vi "Auto Filenames.vi"(8 "Fehler (Eingang)":errorcluster, 9 "Flags Cluster":T4={"PDF Optionen (Eingang)"={"PDF Einzelseiten Komponenten"=FALSE, "PDF Einzelseiten Span"=FALSE, "PDF Deckblatt"=FALSE, "PDF öffnen"=FALSE, "Graphik für Messwerte"=FALSE}, "reprocessing"=FALSE, "1. Komponente"=TRUE, "Pfad AutoLIN in"=path "", "File Name LIN in"="", "Pfad LIN in"=path "", "Filename Overrride"=TRUE}, 10 "Zeitstempel":timestamp, 11 "SpanInletClusterArray in":T9[](array[typedef]) {"zusätzliche Zeitdauer Erster Punkt" min=30 step=1 format="%#_5g"; "Zeitdauer Stufen" format="%#_5g"; "Max Fehler" format="%#_5g"; "Anzahl Stufen" format="%#_5g"; "Komponenten"."Komponente 5"."Komponente:" items=["NO (350,3000) LP 191C", "NO2 (150) LP 191C (1of2)", "NO2 (2000) LP 191C (2of2)", "N2O (300) LP 191C (1of2)", "NH3 (300) LP 191C (1of2)", "NH3 (900,3000) LP 191C (2of2)", "HNCO (400) 191C", "H2O% (30) LP 191C", "Formaldehyde (70,500) LP 191C", "CO2 low% (4) LP 191C (2of2)", "CO2% (20) LP 191C (1of2)", "CO (700) LP 191C (1of3)", "CO% (1) LP 191C (2of3)", "Propylene (1000) LP 191C", "Aromatic HC C7 (500) LP 191C", "Ethylene (1000) LP 191C", "CH4 (250) LP 191C (1of2)", "CH4 (5000) LP 191C (2of2)", "Ethane (1000) LP 191C", "Acetylene (1000) LP 191C", "HNO2 (20) 191C", "MeOH (1000) 191C", "CO% (10) LP 191C (3of3)", "Formic Acid (100) 191C", "SO2 (500) LP 191C", "Acetaldehyde (1000) LP 191C", "COS (100) LP 191C", "1,3 butadiene (100) LP 191C", "Oil as Octane (200) LP 191C", "N2O (1000) LP 191C (2of2)", "Propane (200) LP 191C", "NO2 autorange (2000)", "CO autorange (100000)", "CH4 autorange (5000)", "NH3 autorange (3000)", "Temp. Gascell", "Pressure Gascell", "sBeam@2500"]; "Komponenten"."Komponente 5"."Konzentration IST" format="%#.4f"; "Komponenten"."Komponente 5"."Genauigkeit" format="%#.1f"; "Komponenten"."Komponente 4"."Komponente:" items=["NO (350,3000) LP 191C", "NO2 (150) LP 191C (1of2)", "NO2 (2000) LP 191C (2of2)", "N2O (300) LP 191C (1of2)", "NH3 (300) LP 191C (1of2)", "NH3 (900,3000) LP 191C (2of2)", "HNCO (400) 191C", "H2O% (30) LP 191C", "Formaldehyde (70,500) LP 191C", "CO2 low% (4) LP 191C (2of2)", "CO2% (20) LP 191C (1of2)", "CO (700) LP 191C (1of3)", "CO% (1) LP 191C (2of3)", "Propylene (1000) LP 191C", "Aromatic HC C7 (500) LP 191C", "Ethylene (1000) LP 191C", "CH4 (250) LP 191C (1of2)", "CH4 (5000) LP 191C (2of2)", "Ethane (1000) LP 191C", "Acetylene (1000) LP 191C", "HNO2 (20) 191C", "MeOH (1000) 191C", "CO% (10) LP 191C (3of3)", "Formic Acid (100) 191C", "SO2 (500) LP 191C", "Acetaldehyde (1000) LP 191C", "COS (100) LP 191C", "1,3 butadiene (100) LP 191C", "Oil as Octane (200) LP 191C", "N2O (1000) LP 191C (2of2)", "Propane (200) LP 191C", "NO2 autorange (2000)", "CO autorange (100000)", "CH4 autorange (5000)", "NH3 autorange (3000)", "Temp. Gascell", "Pressure Gascell", "sBeam@2500"]; "Komponenten"."Komponente 4"."Konzentration IST" format="%#.4f"; "Komponenten"."Komponente 4"."Genauigkeit" format="%#.1f"; "Komponenten"."Komponente 3"."Komponente:" items=["NO (350,3000) LP 191C", "NO2 (150) LP 191C (1of2)", "NO2 (2000) LP 191C (2of2)", "N2O (300) LP 191C (1of2)", "NH3 (300) LP 191C (1of2)", "NH3 (900,3000) LP 191C (2of2)", "HNCO (400) 191C", "H2O% (30) LP 191C", "Formaldehyde (70,500) LP 191C", "CO2 low% (4) LP 191C (2of2)", "CO2% (20) LP 191C (1of2)", "CO (700) LP 191C (1of3)", "CO% (1) LP 191C (2of3)", "Propylene (1000) LP 191C", "Aromatic HC C7 (500) LP 191C", "Ethylene (1000) LP 191C", "CH4 (250) LP 191C (1of2)", "CH4 (5000) LP 191C (2of2)", "Ethane (1000) LP 191C", "Acetylene (1000) LP 191C", "HNO2 (20) 191C", "MeOH (1000) 191C", "CO% (10) LP 191C (3of3)", "Formic Acid (100) 191C", "SO2 (500) LP 191C", "Acetaldehyde (1000) LP 191C", "COS (100) LP 191C", "1,3 butadiene (100) LP 191C", "Oil as Octane (200) LP 191C", "N2O (1000) LP 191C (2of2)", "Propane (200) LP 191C", "NO2 autorange (2000)", "CO autorange (100000)", "CH4 autorange (5000)", "NH3 autorange (3000)", "Temp. Gascell", "Pressure Gascell", "sBeam@2500"]; "Komponenten"."Komponente 3"."Konzentration IST" format="%#.4f"; "Komponenten"."Komponente 3"."Genauigkeit" format="%#.1f"; "Komponenten"."Komponente 2"."Komponente:" items=["NO (350,3000) LP 191C", "NO2 (150) LP 191C (1of2)", "NO2 (2000) LP 191C (2of2)", "N2O (300) LP 191C (1of2)", "NH3 (300) LP 191C (1of2)", "NH3 (900,3000) LP 191C (2of2)", "HNCO (400) 191C", "H2O% (30) LP 191C", "Formaldehyde (70,500) LP 191C", "CO2 low% (4) LP 191C (2of2)", "CO2% (20) LP 191C (1of2)", "CO (700) LP 191C (1of3)", "CO% (1) LP 191C (2of3)", "Propylene (1000) LP 191C", "Aromatic HC C7 (500) LP 191C", "Ethylene (1000) LP 191C", "CH4 (250) LP 191C (1of2)", "CH4 (5000) LP 191C (2of2)", "Ethane (1000) LP 191C", "Acetylene (1000) LP 191C", "HNO2 (20) 191C", "MeOH (1000) 191C", "CO% (10) LP 191C (3of3)", "Formic Acid (100) 191C", "SO2 (500) LP 191C", "Acetaldehyde (1000) LP 191C", "COS (100) LP 191C", "1,3 butadiene (100) LP 191C", "Oil as Octane (200) LP 191C", "N2O (1000) LP 191C (2of2)", "Propane (200) LP 191C", "NO2 autorange (2000)", "CO autorange (100000)", "CH4 autorange (5000)", "NH3 autorange (3000)", "Temp. Gascell", "Pressure Gascell", "sBeam@2500"]; "Komponenten"."Komponente 2"."Konzentration IST" format="%#.4f"; "Komponenten"."Komponente 2"."Genauigkeit" format="%#.1f"; "Komponenten"."Komponente 1"."Komponente:" items=["NO (350,3000) LP 191C", "NO2 (150) LP 191C (1of2)", "NO2 (2000) LP 191C (2of2)", "N2O (300) LP 191C (1of2)", "NH3 (300) LP 191C (1of2)", "NH3 (900,3000) LP 191C (2of2)", "HNCO (400) 191C", "H2O% (30) LP 191C", "Formaldehyde (70,500) LP 191C", "CO2 low% (4) LP 191C (2of2)", "CO2% (20) LP 191C (1of2)", "CO (700) LP 191C (1of3)", "CO% (1) LP 191C (2of3)", "Propylene (1000) LP 191C", "Aromatic HC C7 (500) LP 191C", "Ethylene (1000) LP 191C", "CH4 (250) LP 191C (1of2)", "CH4 (5000) LP 191C (2of2)", "Ethane (1000) LP 191C", "Acetylene (1000) LP 191C", "HNO2 (20) 191C", "MeOH (1000) 191C", "CO% (10) LP 191C (3of3)", "Formic Acid (100) 191C", "SO2 (500) LP 191C", "Acetaldehyde (1000) LP 191C", "COS (100) LP 191C", "1,3 butadiene (100) LP 191C", "Oil as Octane (200) LP 191C", "N2O (1000) LP 191C (2of2)", "Propane (200) LP 191C", "NO2 autorange (2000)", "CO autorange (100000)", "CH4 autorange (5000)", "NH3 autorange (3000)", "Temp. Gascell", "Pressure Gascell", "sBeam@2500"]; "Komponenten"."Komponente 1"."Konzentration IST" format="%#.4f"; "Komponenten"."Komponente 1"."Genauigkeit" format="%#.1f"; "Ablaufdatum" format="%<%d.%m.%Y>T"; "Gasflasche" items=["----"=10000, "IAG NH3 3000"=0, "IAG NH3 200"=1, "IAG NH3 2000"=2, "IAG MG"=3, "IAG O2"=4]}) -> (0 "Fehler (Ausgang)":errorcluster, 1 "LogInfo-Cluster":T6 {"Gasflasche" items=["----"=10000, "IAG NH3 3000"=0, "IAG NH3 200"=1, "IAG NH3 2000"=2, "IAG MG"=3, "IAG O2"=4]}, 2 "Pfad LIN Cluster":cluster{"Pfad LIN SPAN":T1, "Pfad LIN":path}, 3 "SpanInletClusterArray out":T9[](array[typedef]) {"zusätzliche Zeitdauer Erster Punkt" min=30 step=1 format="%#_5g"; "Zeitdauer Stufen" format="%#_5g"; "Max Fehler" format="%#_5g"; "Anzahl Stufen" format="%#_5g"; "Komponenten"."Komponente 5"."Komponente:" items=["NO (350,3000) LP 191C", "NO2 (150) LP 191C (1of2)", "NO2 (2000) LP 191C (2of2)", "N2O (300) LP 191C (1of2)", "NH3 (300) LP 191C (1of2)", "NH3 (900,3000) LP 191C (2of2)", "HNCO (400) 191C", "H2O% (30) LP 191C", "Formaldehyde (70,500) LP 191C", "CO2 low% (4) LP 191C (2of2)", "CO2% (20) LP 191C (1of2)", "CO (700) LP 191C (1of3)", "CO% (1) LP 191C (2of3)", "Propylene (1000) LP 191C", "Aromatic HC C7 (500) LP 191C", "Ethylene (1000) LP 191C", "CH4 (250) LP 191C (1of2)", "CH4 (5000) LP 191C (2of2)", "Ethane (1000) LP 191C", "Acetylene (1000) LP 191C", "HNO2 (20) 191C", "MeOH (1000) 191C", "CO% (10) LP 191C (3of3)", "Formic Acid (100) 191C", "SO2 (500) LP 191C", "Acetaldehyde (1000) LP 191C", "COS (100) LP 191C", "1,3 butadiene (100) LP 191C", "Oil as Octane (200) LP 191C", "N2O (1000) LP 191C (2of2)", "Propane (200) LP 191C", "NO2 autorange (2000)", "CO autorange (100000)", "CH4 autorange (5000)", "NH3 autorange (3000)", "Temp. Gascell", "Pressure Gascell", "sBeam@2500"]; "Komponenten"."Komponente 5"."Konzentration IST" format="%#.4f"; "Komponenten"."Komponente 5"."Genauigkeit" format="%#.1f"; "Komponenten"."Komponente 4"."Komponente:" items=["NO (350,3000) LP 191C", "NO2 (150) LP 191C (1of2)", "NO2 (2000) LP 191C (2of2)", "N2O (300) LP 191C (1of2)", "NH3 (300) LP 191C (1of2)", "NH3 (900,3000) LP 191C (2of2)", "HNCO (400) 191C", "H2O% (30) LP 191C", "Formaldehyde (70,500) LP 191C", "CO2 low% (4) LP 191C (2of2)", "CO2% (20) LP 191C (1of2)", "CO (700) LP 191C (1of3)", "CO% (1) LP 191C (2of3)", "Propylene (1000) LP 191C", "Aromatic HC C7 (500) LP 191C", "Ethylene (1000) LP 191C", "CH4 (250) LP 191C (1of2)", "CH4 (5000) LP 191C (2of2)", "Ethane (1000) LP 191C", "Acetylene (1000) LP 191C", "HNO2 (20) 191C", "MeOH (1000) 191C", "CO% (10) LP 191C (3of3)", "Formic Acid (100) 191C", "SO2 (500) LP 191C", "Acetaldehyde (1000) LP 191C", "COS (100) LP 191C", "1,3 butadiene (100) LP 191C", "Oil as Octane (200) LP 191C", "N2O (1000) LP 191C (2of2)", "Propane (200) LP 191C", "NO2 autorange (2000)", "CO autorange (100000)", "CH4 autorange (5000)", "NH3 autorange (3000)", "Temp. Gascell", "Pressure Gascell", "sBeam@2500"]; "Komponenten"."Komponente 4"."Konzentration IST" format="%#.4f"; "Komponenten"."Komponente 4"."Genauigkeit" format="%#.1f"; "Komponenten"."Komponente 3"."Komponente:" items=["NO (350,3000) LP 191C", "NO2 (150) LP 191C (1of2)", "NO2 (2000) LP 191C (2of2)", "N2O (300) LP 191C (1of2)", "NH3 (300) LP 191C (1of2)", "NH3 (900,3000) LP 191C (2of2)", "HNCO (400) 191C", "H2O% (30) LP 191C", "Formaldehyde (70,500) LP 191C", "CO2 low% (4) LP 191C (2of2)", "CO2% (20) LP 191C (1of2)", "CO (700) LP 191C (1of3)", "CO% (1) LP 191C (2of3)", "Propylene (1000) LP 191C", "Aromatic HC C7 (500) LP 191C", "Ethylene (1000) LP 191C", "CH4 (250) LP 191C (1of2)", "CH4 (5000) LP 191C (2of2)", "Ethane (1000) LP 191C", "Acetylene (1000) LP 191C", "HNO2 (20) 191C", "MeOH (1000) 191C", "CO% (10) LP 191C (3of3)", "Formic Acid (100) 191C", "SO2 (500) LP 191C", "Acetaldehyde (1000) LP 191C", "COS (100) LP 191C", "1,3 butadiene (100) LP 191C", "Oil as Octane (200) LP 191C", "N2O (1000) LP 191C (2of2)", "Propane (200) LP 191C", "NO2 autorange (2000)", "CO autorange (100000)", "CH4 autorange (5000)", "NH3 autorange (3000)", "Temp. Gascell", "Pressure Gascell", "sBeam@2500"]; "Komponenten"."Komponente 3"."Konzentration IST" format="%#.4f"; "Komponenten"."Komponente 3"."Genauigkeit" format="%#.1f"; "Komponenten"."Komponente 2"."Komponente:" items=["NO (350,3000) LP 191C", "NO2 (150) LP 191C (1of2)", "NO2 (2000) LP 191C (2of2)", "N2O (300) LP 191C (1of2)", "NH3 (300) LP 191C (1of2)", "NH3 (900,3000) LP 191C (2of2)", "HNCO (400) 191C", "H2O% (30) LP 191C", "Formaldehyde (70,500) LP 191C", "CO2 low% (4) LP 191C (2of2)", "CO2% (20) LP 191C (1of2)", "CO (700) LP 191C (1of3)", "CO% (1) LP 191C (2of3)", "Propylene (1000) LP 191C", "Aromatic HC C7 (500) LP 191C", "Ethylene (1000) LP 191C", "CH4 (250) LP 191C (1of2)", "CH4 (5000) LP 191C (2of2)", "Ethane (1000) LP 191C", "Acetylene (1000) LP 191C", "HNO2 (20) 191C", "MeOH (1000) 191C", "CO% (10) LP 191C (3of3)", "Formic Acid (100) 191C", "SO2 (500) LP 191C", "Acetaldehyde (1000) LP 191C", "COS (100) LP 191C", "1,3 butadiene (100) LP 191C", "Oil as Octane (200) LP 191C", "N2O (1000) LP 191C (2of2)", "Propane (200) LP 191C", "NO2 autorange (2000)", "CO autorange (100000)", "CH4 autorange (5000)", "NH3 autorange (3000)", "Temp. Gascell", "Pressure Gascell", "sBeam@2500"]; "Komponenten"."Komponente 2"."Konzentration IST" format="%#.4f"; "Komponenten"."Komponente 2"."Genauigkeit" format="%#.1f"; "Komponenten"."Komponente 1"."Komponente:" items=["NO (350,3000) LP 191C", "NO2 (150) LP 191C (1of2)", "NO2 (2000) LP 191C (2of2)", "N2O (300) LP 191C (1of2)", "NH3 (300) LP 191C (1of2)", "NH3 (900,3000) LP 191C (2of2)", "HNCO (400) 191C", "H2O% (30) LP 191C", "Formaldehyde (70,500) LP 191C", "CO2 low% (4) LP 191C (2of2)", "CO2% (20) LP 191C (1of2)", "CO (700) LP 191C (1of3)", "CO% (1) LP 191C (2of3)", "Propylene (1000) LP 191C", "Aromatic HC C7 (500) LP 191C", "Ethylene (1000) LP 191C", "CH4 (250) LP 191C (1of2)", "CH4 (5000) LP 191C (2of2)", "Ethane (1000) LP 191C", "Acetylene (1000) LP 191C", "HNO2 (20) 191C", "MeOH (1000) 191C", "CO% (10) LP 191C (3of3)", "Formic Acid (100) 191C", "SO2 (500) LP 191C", "Acetaldehyde (1000) LP 191C", "COS (100) LP 191C", "1,3 butadiene (100) LP 191C", "Oil as Octane (200) LP 191C", "N2O (1000) LP 191C (2of2)", "Propane (200) LP 191C", "NO2 autorange (2000)", "CO autorange (100000)", "CH4 autorange (5000)", "NH3 autorange (3000)", "Temp. Gascell", "Pressure Gascell", "sBeam@2500"]; "Komponenten"."Komponente 1"."Konzentration IST" format="%#.4f"; "Komponenten"."Komponente 1"."Genauigkeit" format="%#.1f"; "Ablaufdatum" format="%<%d.%m.%Y>T"; "Gasflasche" items=["----"=10000, "IAG NH3 3000"=0, "IAG NH3 200"=1, "IAG NH3 2000"=2, "IAG MG"=3, "IAG O2"=4]}, 4 "File Name LIN":T3, 5 "Span_Name":string, 6 "File Name EPA":T3, 7 "File Names":T5)   [LabVIEW 2020, in "Linearisierung v2.lvlib" / "SpanEinstellungen.lvlib"]
uses:
  SpanEinstellungen.lvlib
  Visualisierungs Elemente/String - Eingabefeld.ctl
  SpanInletCluster.ctl
  Seiten/System Einstellungen V2/Konfig Gasflasche.ctl
  Seiten/System Einstellungen V2/Analysatoren.ctl
  Seiten/System Einstellungen V2/Gasflasche Auswahl.ctl
  Komponentencluster mit Formel.ctl
  Komponentenauswahl mit Formel.ctl
  Einheit.ctl
  Seiten/System Einstellungen V2/Traegergas.ctl
  ErrorLogInfoCluster.ctl
  Visualisierungs Elemente/String - Ausgabefeld.ctl
  PDF Optionen.ctl
  Visualisierungs Elemente/Pfad-Eingabefeld.ctl
  Aktion FGV Spans abarbeiten.ctl
  Aktion FGV Post Processing.ctl
  Allgemein/allgemeine Sub-VIs.lvlib
  Seiten/System Einstellungen V2/System Einstellungen V2.lvlib
panel:
  out "Deckblatt LIN":string
  out "Deckblatt EPA":string
  # "sec"
  # "%"
  # "sec"
  # "Komponente"
  # "Formel"
  # "Konzentration"
  # "Einheit"
  # "Genauigkeit [%]"
  # "sec"
  # "%"
  # "sec"
  # "Komponente"
  # "Formel"
  # "Konzentration"
  # "Einheit"
  # "Genauigkeit [%]"
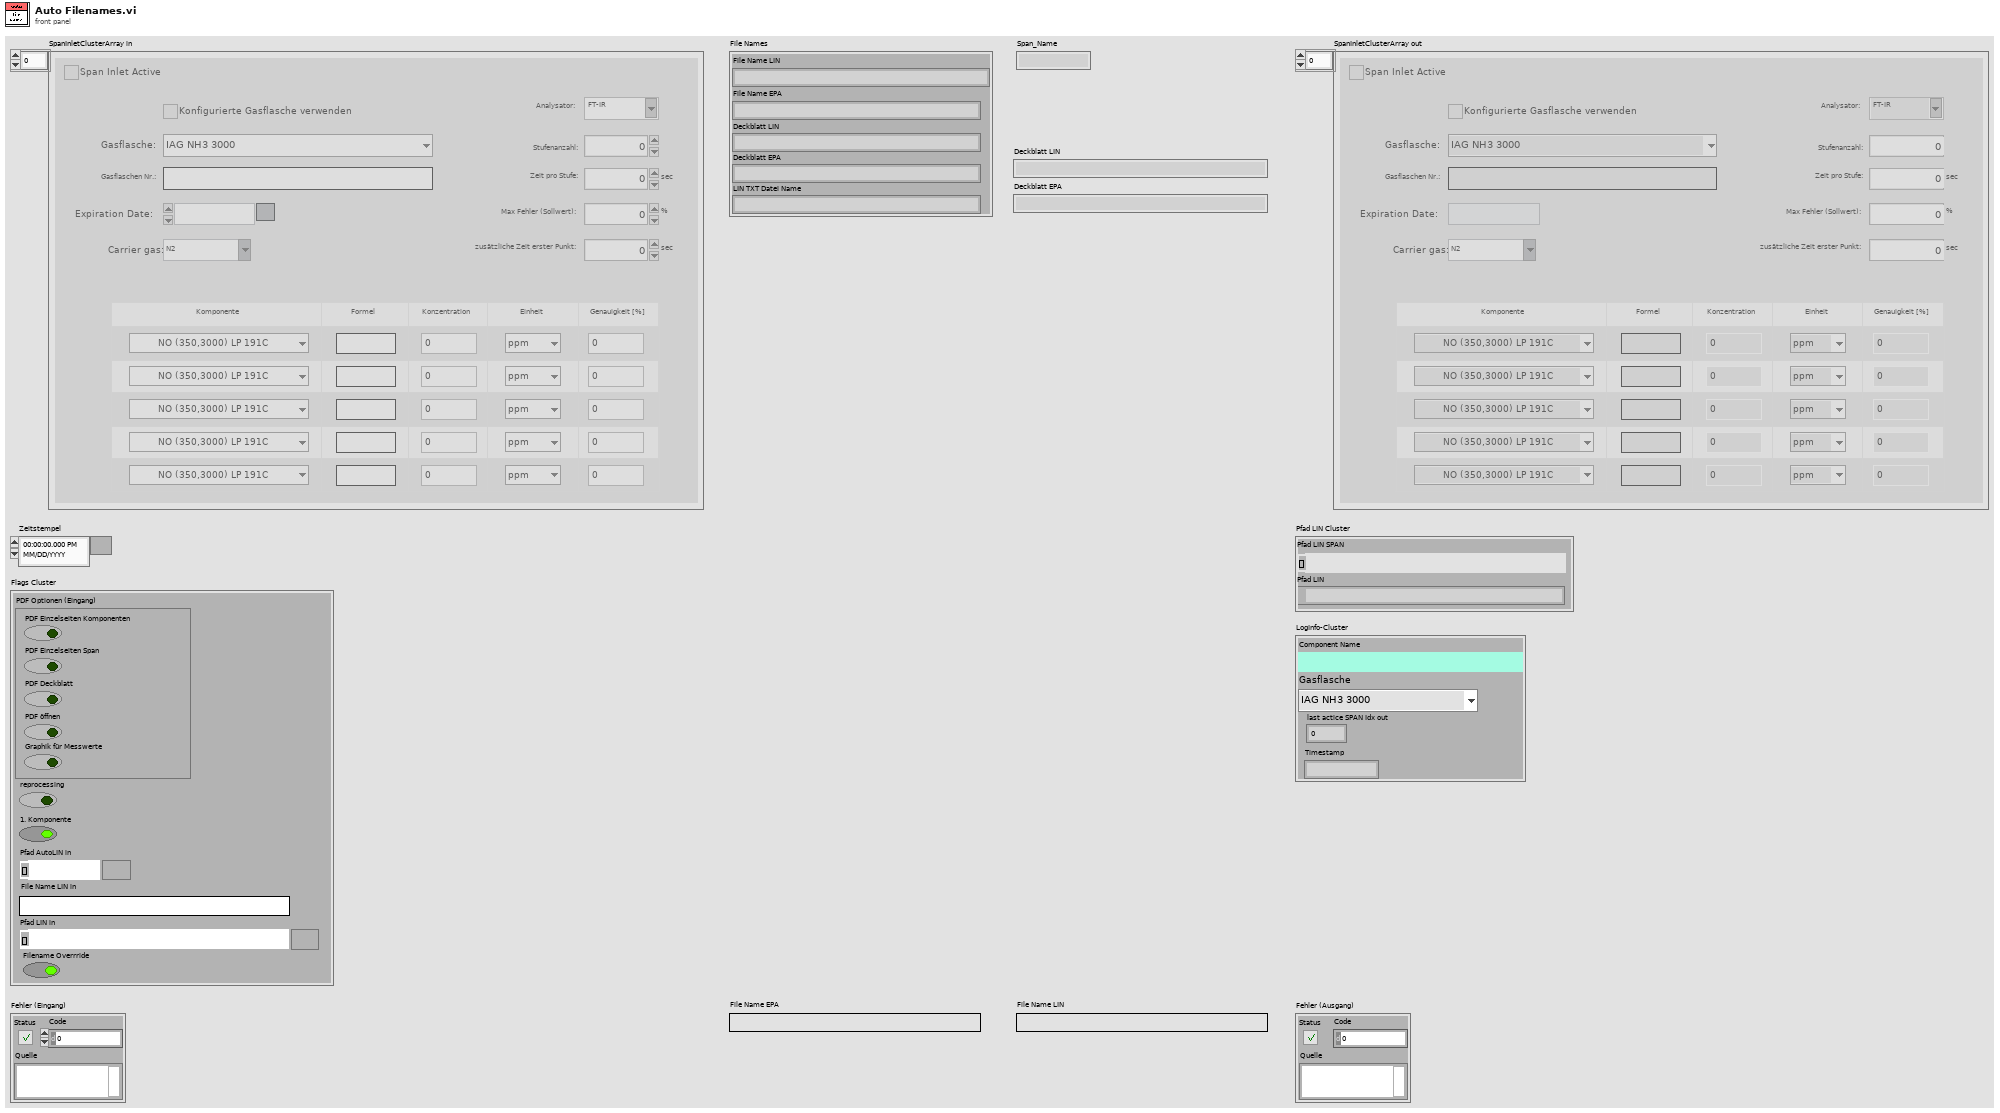
[diagram p1: front panel]
types:
  T1 = typedef "Pfad-Eingabefeld.ctl" = path
  T2 = typedef "Linearisierung v2.lvlib/SpanEinstellungen.lvlib/PDF Optionen.ctl" = cluster{"PDF Einzelseiten Komponenten":bool, "PDF Einzelseiten Span":bool, "PDF Deckblatt":bool, "PDF öffnen":bool, "Graphik für Messwerte":bool}
  T3 = typedef "String - Eingabefeld.ctl" = string
  T4 = cluster{"PDF Optionen (Eingang)":T2, "reprocessing":bool, "1. Komponente":bool, "Pfad AutoLIN in":T1, "File Name LIN in":T3, "Pfad LIN in":T1, "Filename Overrride":bool}
  T5 = cluster{"File Name LIN":string, "File Name EPA":string, "Deckblatt LIN":string, "Deckblatt EPA":string, "LIN TXT Datei Name":string}
  T6 = typedef "Linearisierung v2.lvlib/SpanEinstellungen.lvlib/ErrorLogInfoCluster.ctl" = cluster{"Component Name":T7, "Gasflasche":T8, "last actice SPAN Idx out":i32, "Timestamp":string}
  T7 = typedef "String - Ausgabefeld.ctl" = string
  T8 = typedef "System Einstellungen V2.lvlib/Gasflasche Auswahl.ctl" = u16
  T9 = typedef "Linearisierung v2.lvlib/SpanEinstellungen.lvlib/SpanInletCluster.ctl" = cluster{"Span Inlet Active":T10, "Analysator":T11, "Konfig Gasflasche":T10, "Gasflasche":T8, "Gasflaschen Nr.:":string, "Ablaufdatum":timestamp, "Komponenten":T12, "Zeitdauer Stufen":sgl, "Max Fehler":sgl, "Anzahl Stufen":sgl, "Trägergas":T15, "zusätzliche Zeitdauer Erster Punkt":sgl}
  T10 = typedef "System Einstellungen V2.lvlib/Konfig Gasflasche.ctl" = bool
  T11 = typedef "System Einstellungen V2.lvlib/Analysatoren.ctl" = string
  T12 = typedef "Linearisierung v2.lvlib/SpanEinstellungen.lvlib/Komponentencluster mit Formel.ctl" = cluster{"Komponente 1":T13, "Komponente 2":T13, "Komponente 3":T13, "Komponente 4":T13, "Komponente 5":T13}
  T13 = typedef "Linearisierung v2.lvlib/SpanEinstellungen.lvlib/Komponentenauswahl mit Formel.ctl" = cluster{"Komponente:":u16, "Summenformel":T3, "Konzentration IST":dbl, "Einheit":T14, "Genauigkeit":dbl}
  T14 = typedef "Linearisierung v2.lvlib/SpanEinstellungen.lvlib/Einheit.ctl" = enum16{"ppm", "%"}
  T15 = typedef "System Einstellungen V2.lvlib/Traegergas.ctl" = string
  T16 = typedef "Linearisierung v2.lvlib/SpanEinstellungen.lvlib/Aktion FGV Spans abarbeiten.ctl" = enum16{"lesen", "idle", "start", "next", "comp", "init", "running", "abort"}
  T17 = typedef "Linearisierung v2.lvlib/SpanEinstellungen.lvlib/Aktion FGV Post Processing.ctl" = enum16{"lesen", "set ref", "init", "reset", "enable", "disable", "filenames", "active", "comp", "filename index", "next", "first", "abort", "show", "same"}
  T18 = typedef "Linearisierung v2.lvlib/SpanEinstellungen.lvlib/Postprocessing_Running_Indices.ctl" = cluster{"active postprocessing SPAN":i32, "active postprocessing SPAN Component":i32, "active postprocessing index":i32}
  T19 = cluster{"active Index Cluster out":T18, "last postprocessing SPAN ":bool}
  T20 = cluster{"Component Name":T7, "Compnent Nr":u16, "Formelname(n)":string}
  T21 = cluster{"File Name LIN":string, "File Name EPA":string, "MG":bool}
  T22 = cluster{"Component Name":T7, "Gasflasche":T8, "active postprocessing SPAN":i32, "date/time string":string}
  T23 = cluster{"File Name LIN in":T3, "File Name LIN in":T3, string, string, "File Name LIN":string}
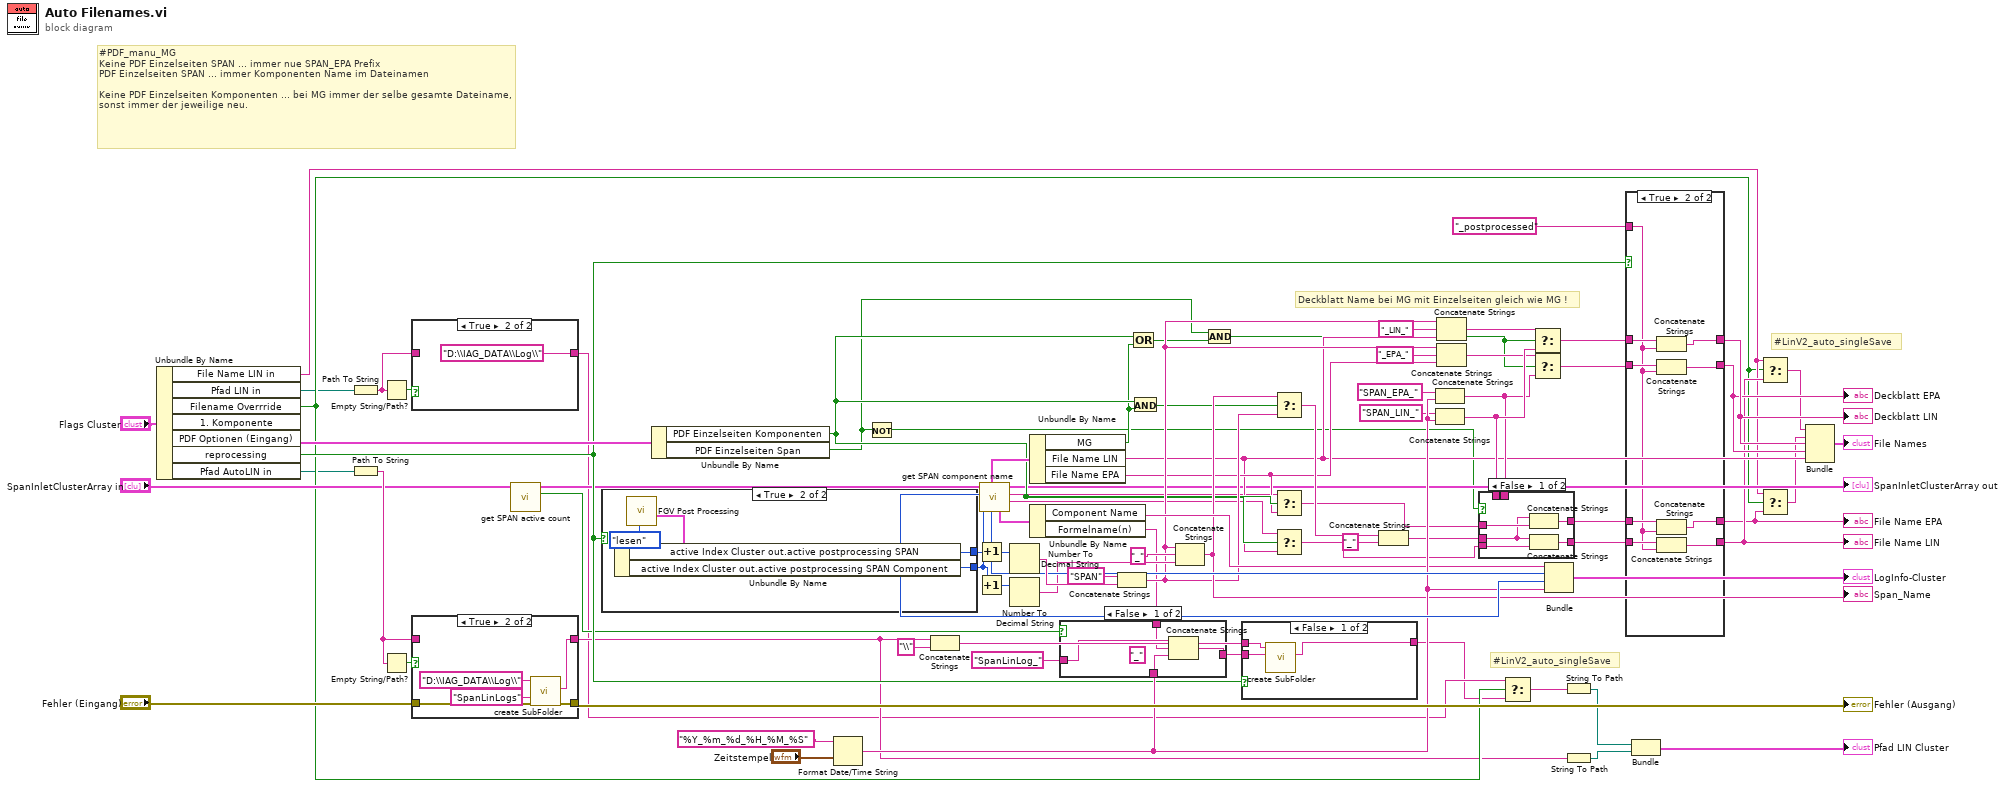
[diagram p0: block diagram]
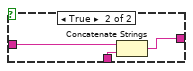
[diagram p4: hidden frame]
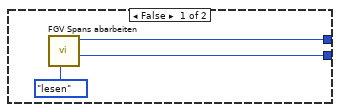
[diagram p6: hidden frame]
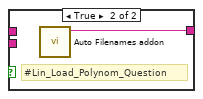
[diagram p7: hidden frame]
diagram:
  # "#LinV2_auto_singleSave"
  # "#LinV2_auto_singleSave"
  # "Deckblatt Name bei MG mit Einzelseiten gleich wie MG !"
  # "#PDF_manu_MG\nKeine PDF Einzelseiten SPAN ... immer nue SPAN_EPA Prefix\nPDF Einzelseiten SPAN ... immer Komponenten Name im Dateinamen\n\nKeine PDF Einzelseiten Komponenten ... bei MG immer der selbe gesamte Dateiname, sonst immer der jeweilige neu."
  n1 = Unbundle By Name("Flags Cluster") -> ("File Name LIN in"=w10:T3, "Pfad LIN in"=w6:T1, "Filename Overrride"=w9:bool, "PDF Optionen (Eingang)"=w63:T2, "reprocessing"=w38:bool, "Pfad AutoLIN in"=w7:T1)  [unwired: 1 out]
  n2 = Path To String(path=w6) -> (string=w4:string)
  n3 = Path To String(path=w7) -> (string=w30:string)
  n4 = Empty String/Path?(string/path=w4) -> (empty?=w5:bool)
  n5 = Empty String/Path?(string/path=w30) -> (empty?=w21:bool)
  n6 = case shown="True" w5 {
    tunnel: w4 -> [w83 _]
    tunnel: [w83 "D:\\IAG_DATA\\Log\\" ("Pfad")] -> w3
    frame False {
    }
    frame True {
    }
  }
  n7 = case shown="True" w21 {
    tunnel: [w85 w91] -> w80
    tunnel: "Fehler (Eingang)" -> [w85 w90]
    tunnel: w30 -> [w86 _]
    tunnel: [w86 w87] -> w8
    frame False {
    }
    frame True {
      n8 = call "create SubFolder.vi"("Fehler (Eingang)"=w90, "Ordner"="SpanLinLogs", "Pfad"="D:\\IAG_DATA\\Log\\") -> ("Fehler (Ausgang)"=w91:errorcluster, "SubOrdner"=w87:string)  [unwired: 6 in, 1 out]
    }
  }
  "Fehler (Ausgang)" <- w80
  n9 = call "get SPAN active count.vi"("SpanInletClusterArray in"="SpanInletClusterArray in") -> ("mehr als 1"=w24:bool, "SpanInletClusterArray out"=w25:T9[])  [unwired: 7 in, 2 out]
  "SpanInletClusterArray out" <- w25
  n10 = case shown="True" w38 {
    tunnel: [w93 w95] -> w76
    tunnel: [w92 w96] -> w71
    frame False {
      n11 = call "FGV Spans abarbeiten.vi"("Aktion"=Aktion_FGV_Spans_abarbeiten."lesen") -> ("Comp Idx out"=w93:i32, "active SPAN Idx out"=w92:i32)  [unwired: 5 in, 4 out]
    }
    frame True {
      n12 = call "FGV Post Processing.vi"("Aktion"=Aktion_FGV_Post_Processing."lesen") -> ("active Index Cluster out"=w98:T19)  [unwired: 7 in, 3 out]
      n13 = Unbundle By Name(w98) -> ("active Index Cluster out.active postprocessing SPAN"=w96:i32, "active Index Cluster out.active postprocessing SPAN Component"=w95:i32)
    }
  }
  n14 = Unbundle By Name(w63) -> ("PDF Einzelseiten Komponenten"=w45:bool, "PDF Einzelseiten Span"=w15:bool)
  n15 = Format Date/Time String(time format string (%c)="%Y_%m_%d_%H_%M_%S" ("Zeitformatierungs-String (%c)"), seconds (now)="Zeitstempel") -> (date/time string=w68:string)  [unwired: 1 in]
  n16 = Not(x=w15) -> (.not. x?=w16:bool)
  n17 = Concatenate Strings(w8, "\\" ("String")) -> (w62:string)
  n18 = Increment(x=w71) -> (x+1=w70:i32)
  n19 = Increment(x=w76) -> (x+1=w69:i32)
  n20 = call "get SPAN component name.vi"("Comp Idx"=w76, "SPAN Idx"=w71, "SpanInletClusterArray in"=w25) -> ("Protokoll Name LIN"=w41:string, "Protokoll Name EPA"=w42:string, "Komponente Nr Name -Cluster"=w75:T20, "Gasflasche"=w74:T8, "LIN/EPA TXT Datei Name"=w59:T21)  [unwired: 1 in, 3 out]
  n21 = Number To Decimal String(number=w70) -> (decimal integer string=w78:string)  [unwired: 1 in]
  n22 = Number To Decimal String(number=w69) -> (decimal integer string=w56:string)  [unwired: 1 in]
  n23 = Unbundle By Name(w59) -> ("MG"=w18:bool, "File Name LIN"=w43:string, "File Name EPA"=w44:string)
  n24 = Unbundle By Name(w75) -> ("Component Name"=w60:T7, "Formelname(n)"=w22:string)
  n25 = case shown="False" w24 {
    tunnel: w68 -> [w102 w105]
    tunnel: [w100 w104] -> w61
    tunnel: "SpanLinLog_" ("Ordner") -> [w101 w103]
    tunnel: w22 -> [w99 _]
    frame False {
      (unwired) "_" ("String")
      n26 = Concatenate Strings(w101, w99, w102) -> (w100:string)
    }
    frame True {
      n27 = Concatenate Strings(w103, w105) -> (w104:string)
    }
  }
  n28 = Concatenate Strings("SPAN" ("String"), w78) -> (w46:string)
  n29 = Or(x=w45, y=w18) -> (x .or. y?=w20:bool)
  n30 = And(x=w45, y=w18) -> (x .and. y?=w19:bool)
  n31 = Concatenate Strings(w46, "_" ("String"), w56) -> (w54:string)
  "Span_Name" <- w54
  n32 = And(x=w15, y=w20) -> (x .and. y?=w17:bool)
  n33 = case shown="False" w38 {
    tunnel: w62 -> [w108 _]
    tunnel: w61 -> [w107 _]
    tunnel: [w106 w109] -> w2
    frame False {
      n34 = call "create SubFolder.vi"("Ordner"=w107, "Pfad"=w108) -> ("SubOrdner"=w106:string)  [unwired: 7 in, 2 out]
    }
    frame True {
      # "#Lin_Load_Polynom_Question"
      n35 = call "Auto Filenames addon.vi"() -> ("SubOrdner"=w109:string)  [unwired: 11 in]
    }
  }
  n36 = Select(t=w54, s=w19, f=w46) -> (s? t:f=w48:string)
  n37 = Select(t=w42, s=w45, f=w44) -> (s? t:f=w40:string)
  n38 = Select(t=w41, s=w45, f=w43) -> (s? t:f=w39:string)
  n39 = Concatenate Strings(w48, "_" ("String")) -> (w55:string)
  n40 = Concatenate Strings("SPAN_EPA_", w68) -> (w47:string)
  n41 = Concatenate Strings("SPAN_LIN_", w68) -> (w53:string)
  n42 = Concatenate Strings(w46, "_LIN_" ("String"), w43) -> (w51:string)
  n43 = Concatenate Strings(w46, "_EPA_" ("String"), w44) -> (w50:string)
  n44 = case shown="False" w16 {
    tunnel: w39 -> [w114 _]
    tunnel: [w113 w115] -> w32
    tunnel: w40 -> [w112 _]
    tunnel: w55 -> [w111 _]
    tunnel: [w110 w116] -> w33
    tunnel: w47 -> [_ w116]
    tunnel: w53 -> [_ w115]
    frame False {
      n45 = Concatenate Strings(w111, w112) -> (w110:string)
      n46 = Concatenate Strings(w111, w114) -> (w113:string)
    }
    frame True {
    }
  }
  n47 = Select(t=w3, s=w9, f=w2) -> (s? t:f=w1:string)
  n48 = Select(t=w51, s=w17, f=w53) -> (s? t:f=w37:string)
  n49 = Select(t=w50, s=w17, f=w47) -> (s? t:f=w36:string)
  n50 = Bundle("Component Name"=w60, "Gasflasche"=w74, "active postprocessing SPAN"=w71, "date/time string"=w68) -> (→"LogInfo-Cluster":T22)  [unwired: 1 in]
  n51 = String To Path(string=w1) -> (path=w28:path)
  n52 = String To Path(string=w8) -> (path=w29:path)
  n53 = case shown="True" w38 {
    tunnel: w37 -> [w120 w129]
    tunnel: w36 -> [w119 w127]
    tunnel: [w120 w128] -> w35
    tunnel: [w119 w126] -> w34
    tunnel: w33 -> [w118 w125]
    tunnel: [w118 w124] -> w12
    tunnel: w32 -> [w117 w123]
    tunnel: [w117 w122] -> w14
    tunnel: "_postprocessed" ("String") -> [_ w121]
    frame False {
    }
    frame True {
      n54 = Concatenate Strings(w129, w121) -> (w128:string)
      n55 = Concatenate Strings(w127, w121) -> (w126:string)
      n56 = Concatenate Strings(w125, w121) -> (w124:string)
      n57 = Concatenate Strings(w123, w121) -> (w122:string)
    }
  }
  "File Name LIN" <- w14
  "File Name EPA" <- w12
  "Deckblatt EPA" <- w34
  "Deckblatt LIN" <- w35
  n58 = Bundle(w28, w29) -> (→"Pfad LIN Cluster":cluster{path, path})  [unwired: 1 in]
  n59 = Select(t=w10, s=w9, f=w14) -> (s? t:f=w13:T3)
  n60 = Select(t=w10, s=w9, f=w12) -> (s? t:f=w11:T3)
  n61 = Bundle("File Name LIN in"=w13, "File Name LIN in"=w11, w35, w34, "File Name LIN"=w43) -> (→"File Names":T23)  [unwired: 1 in]
